vi "DEPRECATED - Avance Auto - David G.vi"(8 "?":i32=127, 9 "Speed Value":dbl, 10 "Drive Motors Name":string="RobotDrive", 11 "Gyro Name":string="RobotDrive") -> ()   [LabVIEW 2017]
uses:
  <vilib>/Rock Robotics/WPI/Utilities/WPI_GetSetVariantRefNum.vi
  <vilib>/Rock Robotics/WPI/RobotDrive/WPI_RobotDriveArcadeDrive_Standard(NoSaturation).vi
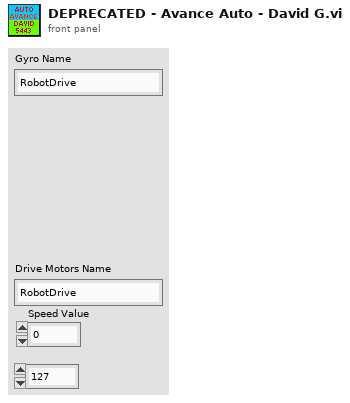
[diagram p1: front panel]
types:
  T1 = typedef "WPI_RobotDriveDevRef.ctl" = cluster{"DevStatus":errorcluster, "Motors[]":T2[], "Square Inputs":bool, "Max Output":dbl}
  T2 = typedef "WPI_MotorControlDeviceRef.ctl" = cluster{"DeviceStatus":errorcluster, "Type":T3, "PWM":cluster{"PWM Channel":T4, "DeadBand":T5}, "CAN":cluster{"Device Number":u8, "SetOutput VI Ref":variant, "GetOutput VI Ref":variant, "Enable VI Ref":variant, "Disable VI Ref":variant, "Data":variant}, "Invert":bool, "DIO PWM":cluster{"PWM \"Enable\" Channel":T4, "DIOChannel":T6, "PWM Rate":dbl}}
  T3 = typedef "WPI_MotorControlType.ctl" = enum16{"PWM", "CAN", "DIO PWM"}
  T4 = typedef "FPGA_DIOPWMChannel.ctl" = enum8{"PWM 0", "PWM 1", "PWM 2", "PWM 3", "PWM 4", "PWM 5", "PWM 6", "PWM 7", "PWM 8", "PWM 9", "PWM MXP 0", "PWM MXP 1", "PWM MXP 2", "PWM MXP 3", "PWM MXP 4", "PWM MXP 5", "PWM MXP 6", "PWM MXP 7", "PWM MXP 8", "PWM MXP 9", "Invalid"}
  T5 = typedef "WPI_PWMDeadband.ctl" = cluster{"Name":string, "maxPositivePwm":i32, "minPositivePwm":i32, "centerPwm":i32, "maxNegativePwm":i32, "minNegativePwm":i32, "angularRange":u16}
  T6 = typedef "FPGA_DIOChannel.ctl" = enum8{"DIO 0", "DIO 1", "DIO 2", "DIO 3", "DIO 4", "DIO 5", "DIO 6", "DIO 7", "DIO 8", "DIO 9", "DIO MXP 0", "DIO MXP 1", "DIO MXP 2", "DIO MXP 3", "DIO MXP 4", "DIO MXP 5", "DIO MXP 6", "DIO MXP 7", "DIO MXP 8", "DIO MXP 9", "DIO MXP 10", "DIO MXP 11", "DIO MXP 12", "DIO MXP 13", "DIO MXP 14", "DIO MXP 15", "SPI Port CS1", "SPI Port CS2", "SPI Port CS3", "SPI Port MISO", "SPI Port MOSI", "Invalid"}
  T7 = typedef "WPI_GyroDevRef.ctl" = cluster{"DevStatus":errorcluster, "Analog Channel":T8, "Gain (VoltsPerDegree/Second)":dbl, "Gyro Type":enum16{"Analog", "XRS450"}, "Handle":i32, "SPI Bus":T9, "Device Found":bool, "Sample Rate":dbl, "Calibrate On Open":bool, "Offset":dbl}
  T8 = typedef "FPGA_AIChannel.ctl" = enum8{"AI 0", "AI 1", "AI 2", "AI 3", "AI MXP 0", "AI MXP 1", "AI MXP 2", "AI MXP 3", "Invalid"}
  T9 = typedef "spi_bus.ctl" = enum16{"SPI On-Board, CS0", "SPI On-Board, CS1", "SPI On-Board, CS2", "SPI On-Board, CS3", "SPI MXP", "Invalid"}
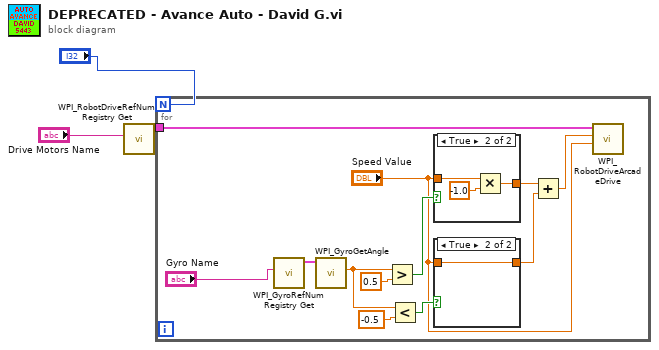
[diagram p0: block diagram]
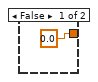
[diagram p2: hidden frame]
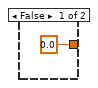
[diagram p3: hidden frame]
diagram:
  n1 = call <vilib>:"WPI_RobotDriveRefNum Registry Get.vi"("refnum name"="Drive Motors Name") -> ("RobotDriveDevRef"=w3:T1)  [unwired: 9 in, 1 out]
  n2 = for {
    N: "?" -> [_]
    tunnel: w3 -> [w15]
    n3 = call <vilib>:"WPI_GyroRefNum Registry Get.vi"("refnum name"="Gyro Name") -> ("GyroDevRef"=w14:T7)  [unwired: 9 in, 1 out]
    n4 = call <vilib>:"WPI_GyroGetAngle.vi"("GyroDevRef"=w14) -> ("Angle"=w12:dbl)  [unwired: 6 in, 4 out]
    n5 = Greater?(x=w12, y=0.5) -> (0:w9:bool)
    n6 = Less?(x=w12, y=-0.5) -> (x < y?=w13:bool)
    n7 = case shown="True" w9 {
      tunnel: [0.0 w21] -> w7
      tunnel: "Speed Value" -> [_ w19]
      frame False {
      }
      frame True {
        n8 = Multiply(x=w19, y=-1.0) -> (x*y=w21:dbl)
      }
    }
    n9 = case shown="True" w13 {
      tunnel: [0.0 w17] -> w8
      tunnel: "Speed Value" -> [_ w17]
      frame False {
      }
      frame True {
      }
    }
    n10 = Add(x=w7, y=w8) -> (x+y=w6:dbl)
    n11 = call-poly <vilib>:"WPI_RobotDriveArcadeDrive.vi"("Y axis value"="Speed Value", "X axis value"=w6, "RobotDriveDevRef"=w15) -> ()  [unwired: 6 in, 3 out]
  }
